vi "Get_7HP_Calib_Info.vi"(0 "Results file":path) -> (1 "ax ay az":sgl[](array[numeric]), 2 "Max Min Yaw":sgl[](array[numeric]), 3 "Max Min Pitch":sgl[](array[numeric]))   [LabVIEW 2022 SP3]
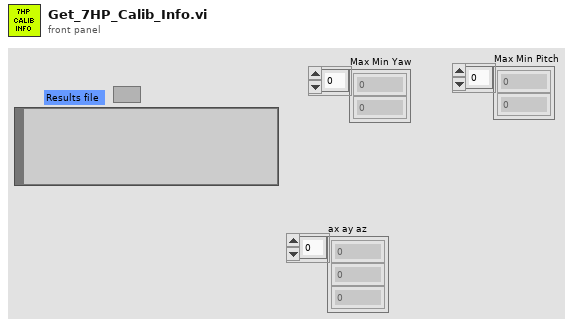
[diagram p1: front panel]
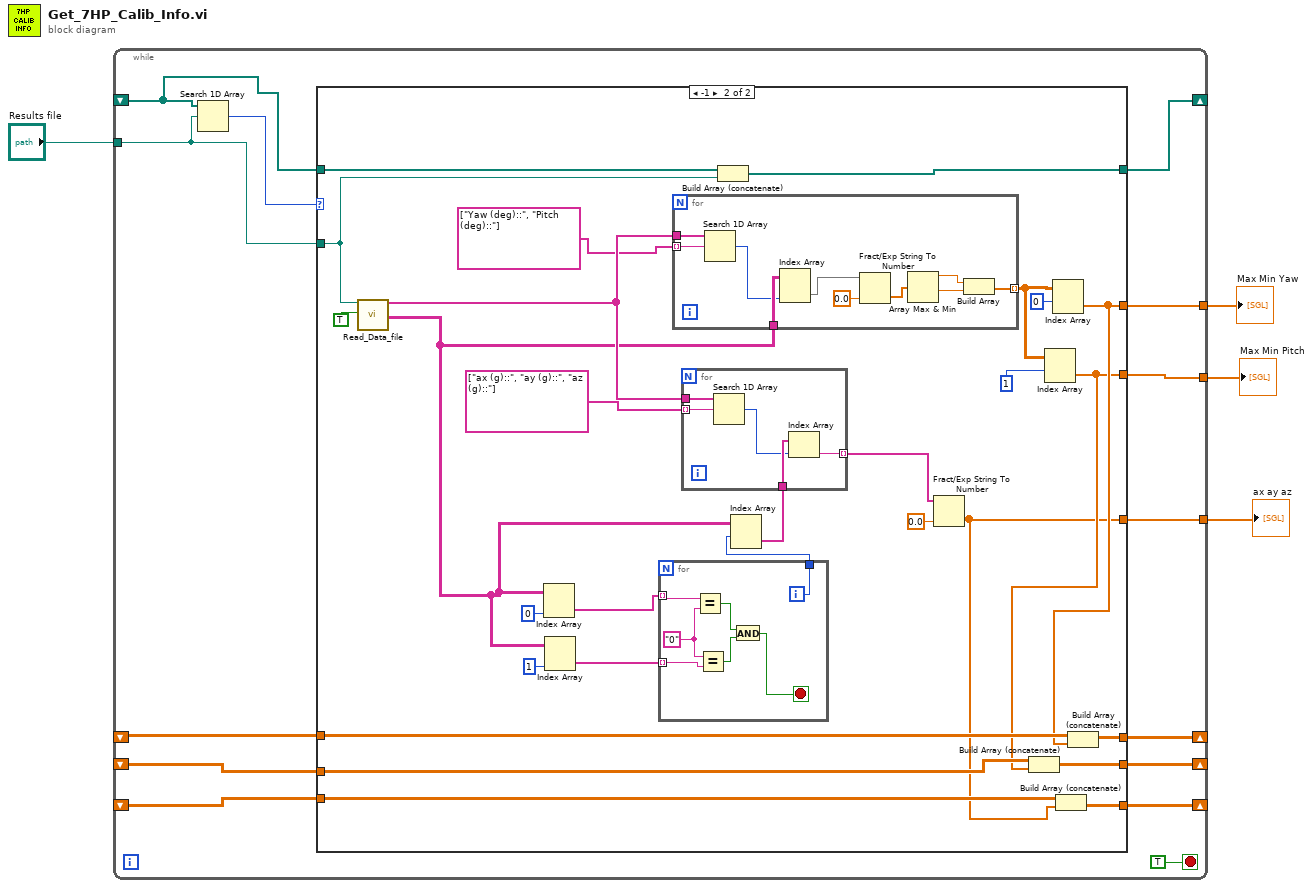
[diagram p0: block diagram]
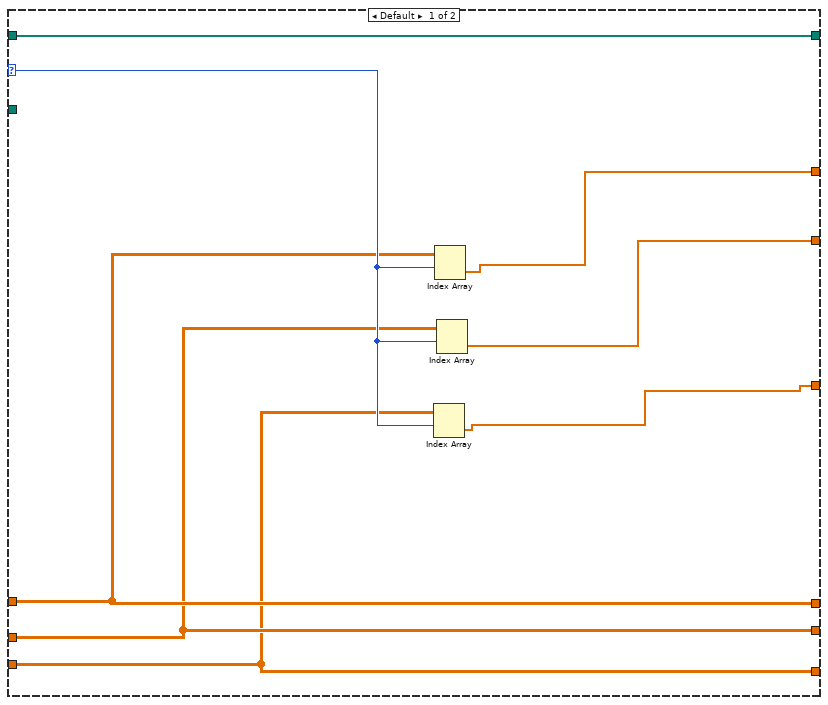
[diagram p2: hidden frame]
diagram:
  n1 = while {
    tunnel: "Results file" -> [w15]
    tunnel: [w18] -> w3
    tunnel: [w17] -> w2
    tunnel: [w16] -> w1
    shift-right: [w13] -> _
    shift-left: _ -> [w12]
    shift-right: [w10] -> _
    shift-left: _ -> [w11]
    shift-right: [w9] -> _
    shift-left: _ -> [w6]
    shift-right: [w8] -> _
    shift-left: _ -> [w7]
    stop <- TRUE stop-if-true
    n2 = Search 1D Array(1D array=w12, element=w15) -> (index of element=w14:i32)  [unwired: 1 in]
    n3 = case shown="-1" w14 {
      selector: w14 -> [w24 _]
      tunnel: w15 -> [_ w37]
      tunnel: [w25 w33] -> w18
      tunnel: [w23 w28] -> w17
      tunnel: [w22 w27] -> w16
      tunnel: [w26 w38] -> w13
      tunnel: w12 -> [w26 w36]
      tunnel: w11 -> [w21 w35]
      tunnel: [w21 w34] -> w10
      tunnel: [w20 w32] -> w9
      tunnel: [w19 w31] -> w8
      tunnel: w7 -> [w19 w30]
      tunnel: w6 -> [w20 w29]
      frame Default {
        n4 = Index Array(array=w19, index (row)=w24) -> (element=w22:sgl[])  [unwired: 1 in]
        n5 = Index Array(array=w21, index (row)=w24) -> (element=w25:sgl[])  [unwired: 1 in]
        n6 = Index Array(array=w20, index (row)=w24) -> (element=w23:sgl[])  [unwired: 1 in]
      }
      frame -1 {
        n7 = call "Read_Data_file.vi"("Results file"=w37, "Delete First Rows?"=TRUE) -> ("Ch names Out"=w44:string[], "Channel Values Out"=w42:string[][])  [unwired: 8 in, 8 out]
        n8 = Index Array(array=w42, index (col)=0 ("disabled index (col)")) -> (element=w50:string[])  [unwired: 1 in]
        n9 = Index Array(array=w42, index (col)=1 ("disabled index (col)")) -> (element=w49:string[])  [unwired: 1 in]
        n10 = for {
          tunnel: w50 -> [w71] mode=indexing
          tunnel: w49 -> [w69] mode=indexing
          tunnel: [w65] -> w48
          i -> [w65]
          stop <- w66 stop-if-true
          w70 = "0" ("element")
          n11 = Equal?(x=w71, y=w70) -> (x = y?=w67:bool)
          n12 = Equal?(x=w70, y=w69) -> (x = y?=w68:bool)
          n13 = And(x=w67, y=w68) -> (x .and. y?=w66:bool)
        }
        n14 = for {
          tunnel: w44 -> [w64]
          tunnel: string[] ["Yaw (deg)::", "Pitch (deg)::"] ("Ch names Out") -> [w63] mode=indexing
          tunnel: w42 -> [w62]
          tunnel: [w55] -> w39 mode=indexing
          n15 = Search 1D Array(1D array=w64, element=w63) -> (index of element=w61:i32)  [unwired: 1 in]
          n16 = Index Array(array=w62, index (col)=w61) -> (element=w59:string[])  [unwired: 1 in]
          n17 = Fract/Exp String To Number(string=w59, default (0 dbl)=sgl 0.0 ("default (0 DBL)")) -> (number=w58:sgl[])  [unwired: 2 in, 1 out]
          n18 = Array Max & Min(array=w58) -> (max value=w56:sgl, min value=w57:sgl)  [unwired: 2 out]
          n19 = Build Array(w56, w57) -> (w55:sgl[])
        }
        n20 = Build Array (concatenate)(w36, w37) -> (w38:path[])
        n21 = Index Array(array=w42, index (row)=w48) -> (element=w47:string[])  [unwired: 1 in]
        n22 = for {
          tunnel: w44 -> [w76]
          tunnel: string[] ["ax (g)::", "ay (g)::", "az (g)::"] ("Ch names Out") -> [w75] mode=indexing
          tunnel: w47 -> [w74]
          tunnel: [w72] -> w46 mode=indexing
          n23 = Search 1D Array(1D array=w76, element=w75) -> (index of element=w73:i32)  [unwired: 1 in]
          n24 = Index Array(array=w74, index=w73) -> (element=w72:string)
        }
        n25 = Fract/Exp String To Number(string=w46, default (0 dbl)=sgl 0.0 ("default (0 DBL)")) -> (number=w27:sgl[])  [unwired: 2 in, 1 out]
        n26 = Index Array(array=w39, index (row)=1) -> (element=w28:sgl[])  [unwired: 1 in]
        n27 = Build Array (concatenate)(w29, w28) -> (w32:sgl[][])
        n28 = Index Array(array=w39, index (row)=0) -> (element=w33:sgl[])  [unwired: 1 in]
        n29 = Build Array (concatenate)(w30, w27) -> (w31:sgl[][])
        n30 = Build Array (concatenate)(w35, w33) -> (w34:sgl[][])
      }
    }
  }
  "Max Min Yaw" <- w3
  "Max Min Pitch" <- w2
  "ax ay az" <- w1
